vi "string-attribute-to-dll-format.vi"(10 "values":string[](array[string]), 11 "keys":string[](array[string])) -> (0 "values_length":i32[](array[numeric]), 1 "values":i8[](array[numeric]), 2 "keys_length":i32[](array[numeric]), 3 "keys":i8[](array[numeric]), 5 "attribute count":i32)   [LabVIEW 2011, in "librir.lvlib"]
uses:
  librir.lvlib
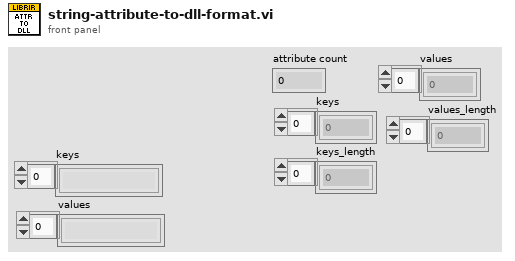
[diagram p1: front panel]
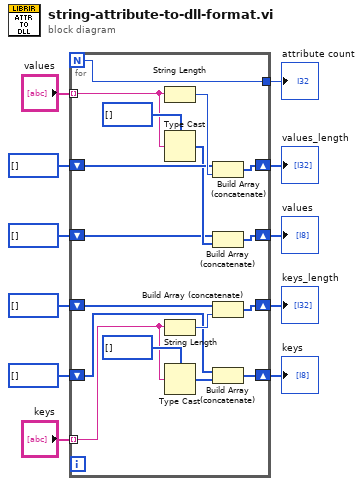
[diagram p0: block diagram]
diagram:
  n1 = for {
    N -> [w12]
    tunnel: "values" -> [w27] mode=indexing
    tunnel: "keys" -> [w17] mode=indexing
    shift-right: [w25] -> w1
    shift-left: i32[] [] -> [w24]
    shift-right: [w22] -> w9
    shift-left: i8[] [] -> [w21]
    shift-right: [w16] -> w6
    shift-left: i32[] [] -> [w15]
    shift-right: [w14] -> w5
    shift-left: i8[] [] -> [w13]
    tunnel: [w12] -> w4
    n2 = String Length(string=w27) -> (length=w26:i32)
    n3 = Type Cast(type=i8[] [] ("keys"), x=w27) -> (*(type *) &x=w23:i8[])
    n4 = String Length(string=w17) -> (length=w19:i32)
    n5 = Type Cast(type=i8[] [] ("keys"), x=w17) -> (*(type *) &x=w20:i8[])
    n6 = Build Array (concatenate)(w24, w26) -> (w25:i32[])
    n7 = Build Array (concatenate)(w21, w23) -> (w22:i8[])
    n8 = Build Array (concatenate)(w15, w19) -> (w16:i32[])
    n9 = Build Array (concatenate)(w13, w20) -> (w14:i8[])
  }
  "attribute count" <- w4
  "keys" <- w5
  "keys_length" <- w6
  "values" <- w9
  "values_length" <- w1
